vi "create_module_map.vi"(11 "variable_info_in":T2) -> (3 "IO_variable_map":T1[](array[typedef]))   [LabVIEW 2015, in "Scan Engine runtime.lvclass"]
uses:
  Scan Engine runtime.lvclass
  Custom Ctrls/Index Map.ctl
  <vilib>/NI/Tag Bus/tag/Data Type.ctl
  Custom Ctrls/IO_index_map.ctl
  <vilib>/NI/Tag Bus/tag/tag descriptor.lvclass
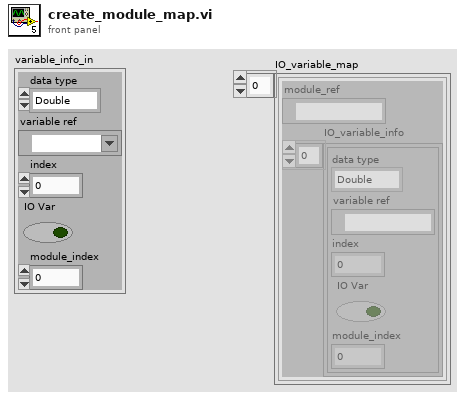
[diagram p1: front panel]
types:
  T1 = typedef "IO_index_map.ctl" = cluster{"module_ref":refnum<k21>, "IO_variable_info":T2[]}
  T2 = typedef "Scan Engine runtime.lvclass/Index Map.ctl" = cluster{"data type":T3, "variable ref":refnum<k21>, "index":i32, "IO Var":bool, "module_index":i32}
  T3 = typedef "tag bus.lvlib/tag descriptor.lvclass/Data Type.ctl" = enum16{"Double", "Single", "I64", "I32", "I16", "I8", "U64", "U32", "U16", "U8", "Boolean", "String", "Array of Double", "Array of Single", "Array of I64", "Array of I32", "Array of I16", "Array of I8", "Array of U64", "Array of U32", "Array of U16", "Array of U8", "Array of Boolean", "Array of String"}
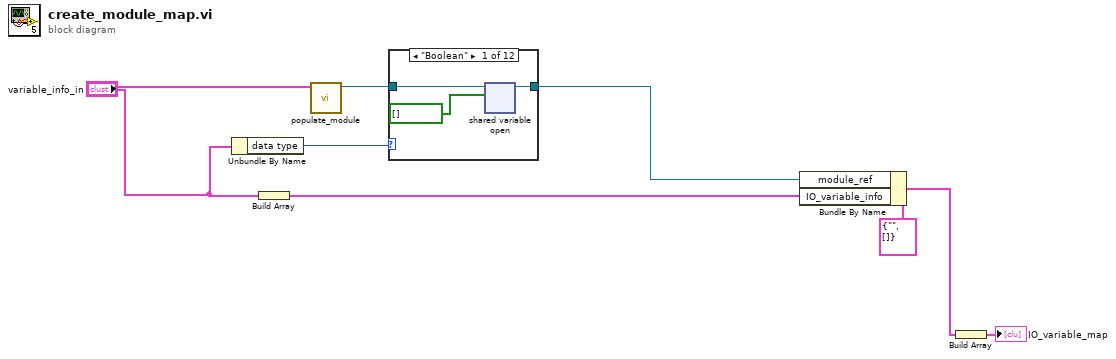
[diagram p0: block diagram]
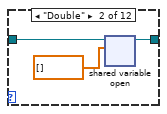
[diagram p2: hidden frame]
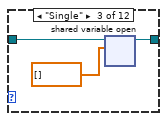
[diagram p3: hidden frame]
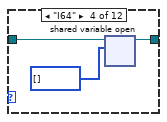
[diagram p4: hidden frame]
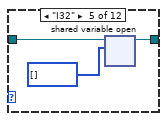
[diagram p5: hidden frame]
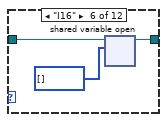
[diagram p6: hidden frame]
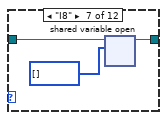
[diagram p7: hidden frame]
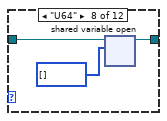
[diagram p8: hidden frame]
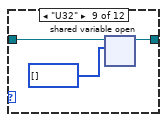
[diagram p9: hidden frame]
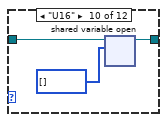
[diagram p10: hidden frame]
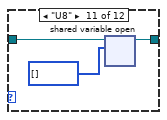
[diagram p11: hidden frame]
diagram:
  n1 = Unbundle By Name("variable_info_in") -> ("data type"=w1:T3)
  n2 = Build Array("variable_info_in") -> (w7:T2[])
  n3 = call "populate_module.vi"("variable_info_in"="variable_info_in") -> ("Module"=w3:refnum<k21>)  [unwired: 10 in]
  n4 = case shown="\"Boolean\"" w1 {
    tunnel: [w9 w12 w15 w19 w21 w24 w27 w30 w33 w36 w39 w42] -> w2
    tunnel: w3 -> [w11 w14 w17 w20 w23 w26 w29 w32 w35 w38 w41 w42]
    frame "Boolean" {
      n5 = shared-variable-open(w11, bool[] []) -> (w9:refnum<k21>)  [unwired: 1 in, 1 out]
    }
    frame "Double" {
      n6 = shared-variable-open(w14, dbl[] []) -> (w12:refnum<k21>)  [unwired: 1 in, 1 out]
    }
    frame "Single" {
      n7 = shared-variable-open(w17, sgl[] []) -> (w15:refnum<k21>)  [unwired: 1 in, 1 out]
    }
    frame "I64" {
      n8 = shared-variable-open(w20, i64[] []) -> (w19:refnum<k21>)  [unwired: 1 in, 1 out]
    }
    frame "I32" {
      n9 = shared-variable-open(w23, i32[] []) -> (w21:refnum<k21>)  [unwired: 1 in, 1 out]
    }
    frame "I16" {
      n10 = shared-variable-open(w26, i16[] []) -> (w24:refnum<k21>)  [unwired: 1 in, 1 out]
    }
    frame "I8" {
      n11 = shared-variable-open(w29, i8[] []) -> (w27:refnum<k21>)  [unwired: 1 in, 1 out]
    }
    frame "U64" {
      n12 = shared-variable-open(w32, u64[] []) -> (w30:refnum<k21>)  [unwired: 1 in, 1 out]
    }
    frame "U32" {
      n13 = shared-variable-open(w35, u32[] []) -> (w33:refnum<k21>)  [unwired: 1 in, 1 out]
    }
    frame "U16" {
      n14 = shared-variable-open(w38, u16[] []) -> (w36:refnum<k21>)  [unwired: 1 in, 1 out]
    }
    frame "U8" {
      n15 = shared-variable-open(w41, u8[] []) -> (w39:refnum<k21>)  [unwired: 1 in, 1 out]
    }
    frame "String", Default {
    }
  }
  n16 = Bundle By Name(cluster=T1 {"module_ref"="", "IO_variable_info"=[]} ("IO_variables_per_module"), "module_ref"=w2, "IO_variable_info"=w7) -> (w8:T1)
  n17 = Build Array(w8) -> (→"IO_variable_map":T1[])
